vi "Open Lead Falcon.vi"(5 "refnum name":string="TalonSRX", 6 "Supply Current Limit Configuration":T1, 7 "PIDF Constants":T2, 8 "error in (no error)":errorcluster, 9 "Drive Sensor Phase":bool, 10 "Drive Invert":bool, 11 "can id":u8) -> (0 "error out":errorcluster, 3 "PhoenixMotorControlDevRef":T3={"DeviceStatus"={"status"=FALSE, "code"=0, "source"=""}, "Type"=enum."PWM", "PWM"={"PWM Channel"=enum."Invalid", "DeadBand"={"Name"="", "maxPositivePwm"=0, "minPositivePwm"=0, "centerPwm"=0, "maxNegativePwm"=0, "minNegativePwm"=0, "angularRange"=0}}, "CAN"={"Device Number"=0, "SetOutput VI Ref"=variant(refnum<vi> refnum), "GetOutput VI Ref"=variant(refnum<vi> refnum), "Enable VI Ref"=variant(refnum<vi> refnum), "Disable VI Ref"=variant(refnum<vi> refnum), "Data"=variant}, "Invert"=FALSE, "DIO PWM"={"PWM \"Enable\" Channel"=enum."Invalid", "DIOChannel"=enum."Invalid", "PWM Rate"=0.0}})   [LabVIEW 2019, in "Climber.lvlib" / "Climber.lvclass"]
uses:
  Climber.lvclass
  <vilib>/Rock Robotics/WPI/MotorControl/WPI_MotorControlDeviceRef.ctl
  <vilib>/Rock Robotics/WPI/MotorControl/WPI_MotorControlType.ctl
  <vilib>/Rock Robotics/SystemInterfaces/DIO/FPGA_DIOPWMChannel.ctl
  <vilib>/Rock Robotics/WPI/PWM/WPI_PWMDeadband.ctl
  <vilib>/Rock Robotics/SystemInterfaces/DIO/FPGA_DIOChannel.ctl
  Drive/Tank Drive/Controls/PIDF.ctl
  <vilib>/Rock Robotics/WPI/ThirdParty/Phoenix-LabVIEW/Motor Controller/Controls/CTRE_Phoenix_MotorControl_SupplyCurrentLimitConfiguration.ctl
  <vilib>/Rock Robotics/WPI/ThirdParty/Phoenix-LabVIEW/Motor Controller/Controls/CTRE_Phoenix_MotorControl_FeedbackDevice_TalonFX.ctl
  <vilib>/Rock Robotics/WPI/ThirdParty/Phoenix-LabVIEW/Motor Controller/Controls/CTRE_Phoenix_MotorControl_TalonFXInvertType.ctl
  Drive/Tank Drive/Tank Drive.lvclass
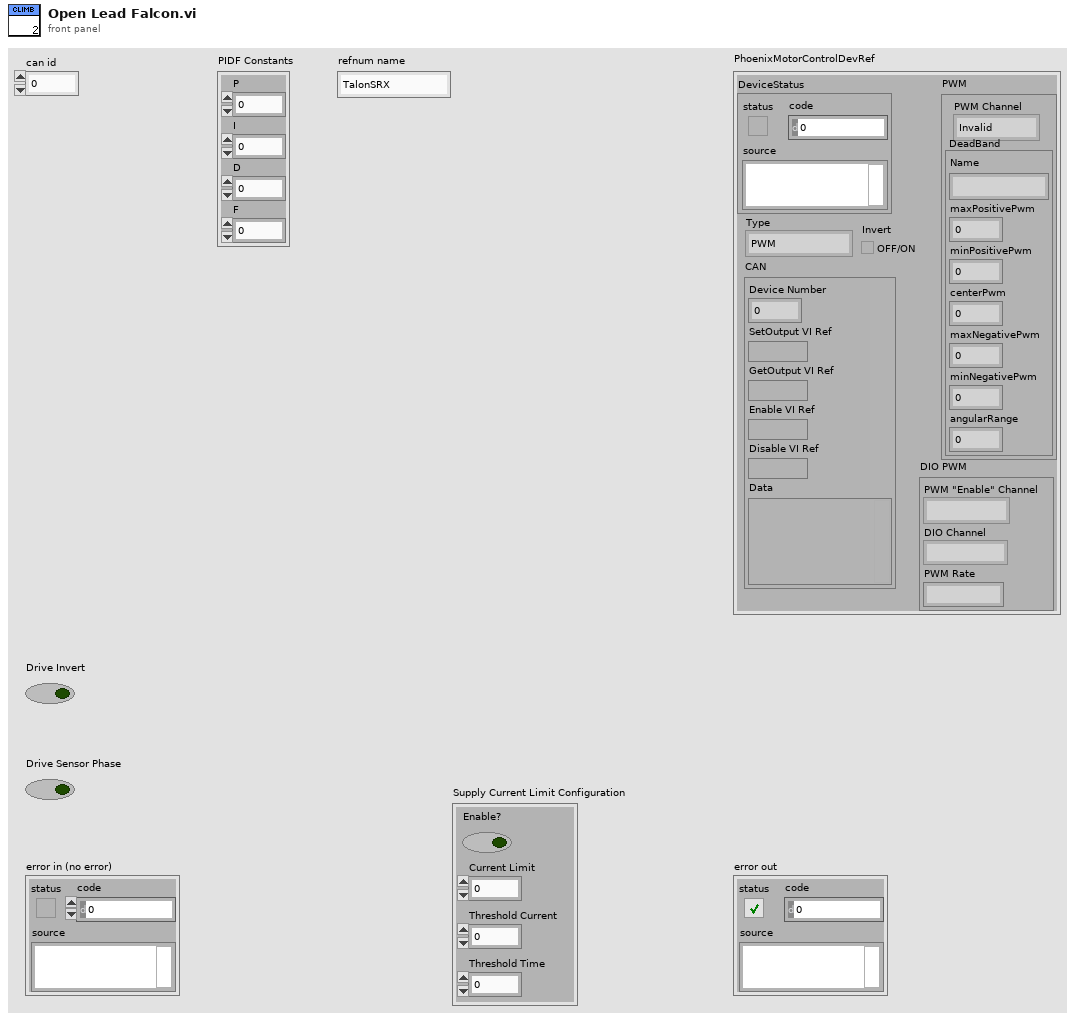
[diagram p1: front panel]
types:
  T1 = typedef "CTRE_Phoenix_MotorControl_SupplyCurrentLimitConfiguration.ctl" = cluster{"Enable?":bool, "Current Limit":dbl, "Threshold Current":dbl, "Threshold Time":dbl}
  T2 = typedef "Drive.lvlib/Tank Drive.lvclass/PIDF.ctl" = cluster{"P":dbl, "I":dbl, "D":dbl, "F":dbl}
  T3 = typedef "WPI_MotorControlDeviceRef.ctl" = cluster{"DeviceStatus":errorcluster, "Type":T4, "PWM":cluster{"PWM Channel":T5, "DeadBand":T6}, "CAN":cluster{"Device Number":u8, "SetOutput VI Ref":variant, "GetOutput VI Ref":variant, "Enable VI Ref":variant, "Disable VI Ref":variant, "Data":variant}, "Invert":bool, "DIO PWM":cluster{"PWM \"Enable\" Channel":T5, "DIOChannel":T7, "PWM Rate":dbl}}
  T4 = typedef "WPI_MotorControlType.ctl" = enum16{"PWM", "CAN", "DIO PWM"}
  T5 = typedef "FPGA_DIOPWMChannel.ctl" = enum8{"PWM 0", "PWM 1", "PWM 2", "PWM 3", "PWM 4", "PWM 5", "PWM 6", "PWM 7", "PWM 8", "PWM 9", "PWM MXP 0", "PWM MXP 1", "PWM MXP 2", "PWM MXP 3", "PWM MXP 4", "PWM MXP 5", "PWM MXP 6", "PWM MXP 7", "PWM MXP 8", "PWM MXP 9", "Invalid"}
  T6 = typedef "WPI_PWMDeadband.ctl" = cluster{"Name":string, "maxPositivePwm":i32, "minPositivePwm":i32, "centerPwm":i32, "maxNegativePwm":i32, "minNegativePwm":i32, "angularRange":u16}
  T7 = typedef "FPGA_DIOChannel.ctl" = enum8{"DIO 0", "DIO 1", "DIO 2", "DIO 3", "DIO 4", "DIO 5", "DIO 6", "DIO 7", "DIO 8", "DIO 9", "DIO MXP 0", "DIO MXP 1", "DIO MXP 2", "DIO MXP 3", "DIO MXP 4", "DIO MXP 5", "DIO MXP 6", "DIO MXP 7", "DIO MXP 8", "DIO MXP 9", "DIO MXP 10", "DIO MXP 11", "DIO MXP 12", "DIO MXP 13", "DIO MXP 14", "DIO MXP 15", "SPI Port CS1", "SPI Port CS2", "SPI Port CS3", "SPI Port MISO", "SPI Port MOSI", "Invalid"}
  T8 = typedef "CTRE_Phoenix_MotorControl_FeedbackDevice_TalonFX.ctl" = i8
  T9 = typedef "CTRE_Phoenix_MotorControl_TalonFXInvertType.ctl" = enum16{"Counter-Clockwise", "Clockwise"}
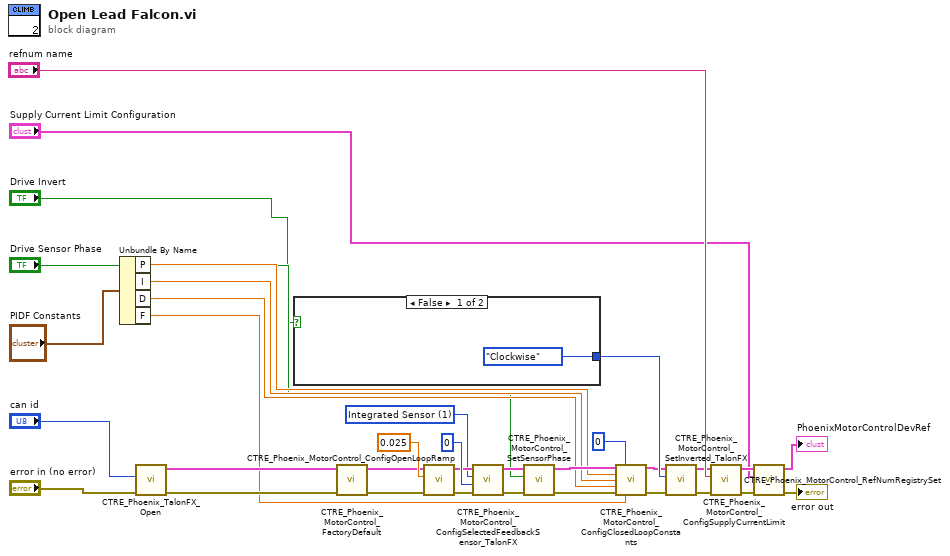
[diagram p0: block diagram]
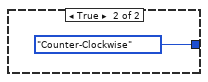
[diagram p2: hidden frame]
diagram:
  w13 = T8 1 items=["Integrated Sensor"=1, "Sensor Sum (S0 + S1)"=9, "Sensor Difference (D0 - D1)"=10, "Remote Source 0"=11, "Remote Source 1"=12, "None"=14, "Software Emulated"=15] ("Talon FX Feedback Device")
  n1 = Unbundle By Name("PIDF Constants") -> ("P"=w7:dbl, "I"=w6:dbl, "D"=w5:dbl, "F"=w4:dbl)
  n2 = call <vilib>:"CTRE_Phoenix_TalonFX_Open.vi"("error in"="error in (no error)", "Device Number"="can id") -> ("error out"=w31:errorcluster, "CAN Talon SRX Ref"=w30:T3)  [unwired: 8 in]
  n3 = case shown="False" "Drive Invert" {
    tunnel: [CTRE_Phoenix_MotorControl_TalonFXInvertType."Clockwise" ("Invert Type") CTRE_Phoenix_MotorControl_TalonFXInvertType."Counter-Clockwise" ("Invert Type")] -> w19
    frame False {
    }
    frame True {
    }
  }
  n4 = call <vilib>:"CTRE_Phoenix_MotorControl_FactoryDefault.vi"("error in"=w31, "PhoenixMotorControlDevRef"=w30) -> ("error out"=w24:errorcluster, "PhoenixMotorControlDevRef"=w25:T3)  [unwired: 8 in]
  n5 = call <vilib>:"CTRE_Phoenix_MotorControl_ConfigOpenLoopRamp.vi"("error in (no error)"=w24, "secondsFromNeutralToFull"=0.025, "PhoenixMotorControlDevRef"=w25) -> ("error out"=w22:errorcluster, "PhoenixMotorControlDevRef"=w23:T3)  [unwired: 7 in]
  n6 = call <vilib>:"CTRE_Phoenix_MotorControl_ConfigSelectedFeedbackSensor_TalonFX.vi"("error in (no error)"=w22, "pidLoopIdx"=0, "Talon FX Feedback Device"=w13, "PhoenixMotorControlDevRef"=w23) -> ("error out"=w27:errorcluster, "PhoenixMotorControlDevRef"=w28:T3)  [unwired: 6 in]
  n7 = call <vilib>:"CTRE_Phoenix_MotorControl_SetSensorPhase.vi"("error in (no error)"=w27, "PhaseSensor"="Drive Sensor Phase", "PhoenixMotorControlDevRef"=w28) -> ("error out"=w17:errorcluster, "PhoenixMotorControlDevRef"=w18:T3)  [unwired: 7 in]
  n8 = call <vilib>:"CTRE_Phoenix_MotorControl_ConfigClosedLoopConstants.vi"("PhoenixMotorControlDevRef"=w18, "slotIdx"=0, "P"=w7, "I"=w6, "D"=w5, "error in (no error)"=w17, "F"=w4) -> ("PhoenixMotorControlDevRef"=w16:T3, "error out"=w15:errorcluster)  [unwired: 7 in]
  n9 = call <vilib>:"CTRE_Phoenix_MotorControl_SetInverted_TalonFX.vi"("error in (no error)"=w15, "Invert Type"=w19, "PhoenixMotorControlDevRef"=w16) -> ("error out"=w21:errorcluster, "PhoenixMotorControlDevRef"=w20:T3)  [unwired: 7 in]
  n10 = call <vilib>:"CTRE_Phoenix_MotorControl_RefNumRegistrySet.vi"("error in (no error)"=w21, "refnum name"="refnum name", "PhoenixMotorControlDevRef"=w20) -> ("error out"=w10:errorcluster, "PhoenixMotorControlDevRef"=w12:T3)  [unwired: 7 in]
  n11 = call <vilib>:"CTRE_Phoenix_MotorControl_ConfigSupplyCurrentLimit.vi"("error in (no error)"=w10, "Supply Current Limit Configuration"="Supply Current Limit Configuration", "PhoenixMotorControlDevRef"=w12) -> ("error out"=→"error out":errorcluster, "PhoenixMotorControlDevRef"=→"PhoenixMotorControlDevRef":T3)  [unwired: 7 in]
